vi "WiFi HttpsPOST.vi"   [LabVIEW 2014]
uses:
  <vilib>/Aledyne-TSXperts/Arduino Compatible Compiler for LabVIEW/Code Generator/Arduino APIs/Digital/PinDirection.ctl
  QwaveSys_ESP8266/QwaveSys_ESP8266.lvlib
  <vilib>/Aledyne-TSXperts/Arduino Compatible Compiler for LabVIEW/Arduino Compatible Compiler for LabVIEW.lvlib
types:
  T1 = typedef "Arduino Compatible Compiler for LabVIEW.lvlib/PinDirection.ctl" = enum16{" INPUT", "OUTPUT", " INPUT_PULLUP"}
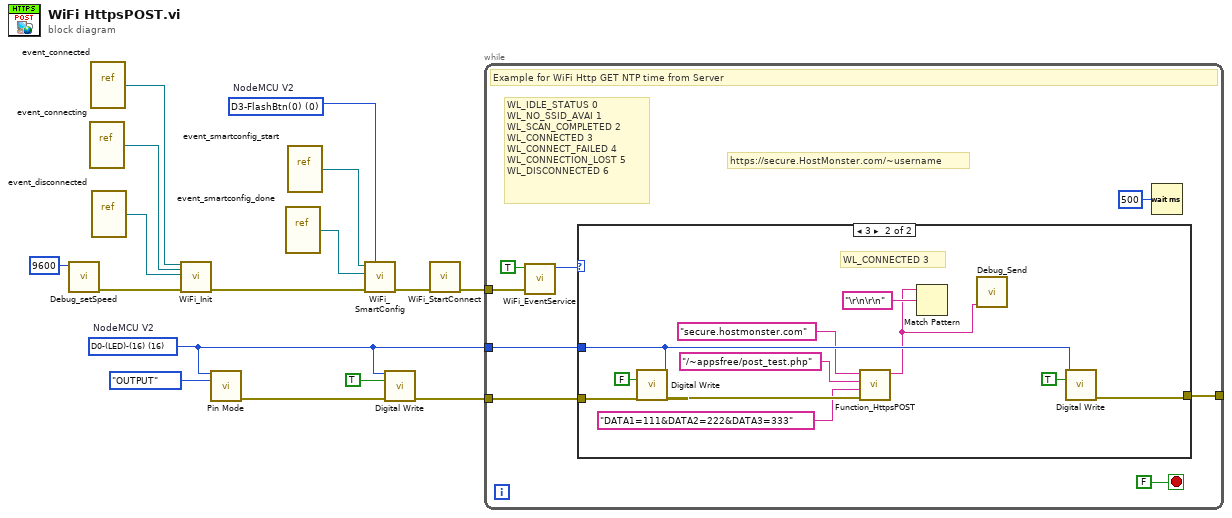
[diagram p0: block diagram]
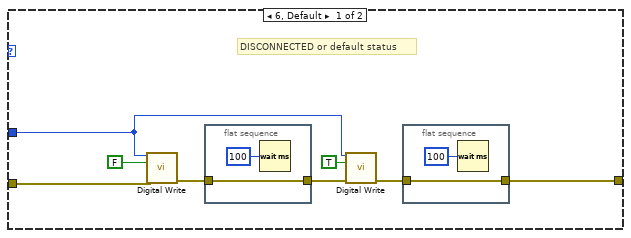
[diagram p2: hidden frame]
diagram:
  w2 = u8 16 items=["D0-(LED)-(16)"=16, "D1-SCL(5)"=5, "D2-SDA(4)"=4, "D3-FlashBtn(0)"=0, "D4-(2)"=2, "D5-SCK(14)"=14, "D6-MISO(12)"=12, "D7-MOSI(13)"=13, "D8-SS(15)"=15, "D9-TX(3)"=3, "D10-RX(1)"=1, "ADC0,(17)"=17]  # NodeMCU V2
  w1 = u8 0 items=["D0-(LED)-(16)"=16, "D1-SCL(5)"=5, "D2-SDA(4)"=4, "D3-FlashBtn(0)"=0, "D4-(2)"=2, "D5-SCK(14)"=14, "D6-MISO(12)"=12, "D7-MOSI(13)"=13, "D8-SS(15)"=15, "D9-TX(3)"=3, "D10-RX(1)"=1, "ADC0,(17)"=17]  # NodeMCU V2
  n1 = call "Debug_setSpeed.vi"("Speed"=u32 9600) -> ("error out"=w8:errorcluster)  [unwired: 10 in]
  n2 = vi-ref "event_connecting.vi"() -> (w13:refnum<vi>)
  n3 = vi-ref "event_connected.vi"() -> (w12:refnum<vi>)
  n4 = vi-ref "event_disconnected.vi"() -> (w11:refnum<vi>)
  n5 = call "WiFi_Init.vi"("connected"=w12, "connecting"=w13, "disconnected"=w11, "error in (no error)"=w8) -> ("error out"=w16:errorcluster)  [unwired: 11 in]
  n6 = call <vilib>:"Pin Mode.vi"("pin"=w2, "direction"=PinDirection."OUTPUT" ("Direction")) -> ("error out"=w4:errorcluster)  [unwired: 13 in]
  n7 = vi-ref "event_smartconfig_done.vi"() -> (w9:refnum<vi>)
  n8 = vi-ref "event_smartconfig_start.vi"() -> (w10:refnum<vi>)
  n9 = call "WiFi_SmartConfig.vi"("Smart Config Enter Pin"=w1, "error in (no error)"=w16, "smartconfig_done"=w9, "smartconfig_start"=w10) -> ("error out"=w15:errorcluster)  [unwired: 7 in]
  n10 = call <vilib>:"Digital Write.vi"("pin"=w2, "state"=TRUE, "error in (no error)"=w4) -> ("error out"=w3:errorcluster)  [unwired: 12 in]
  n11 = call "WiFi_StartConnect.vi"("error in (no error)"=w15) -> ("error out"=w14:errorcluster)  [unwired: 10 in]
  n12 = while {
    tunnel: w14 -> [w23]
    tunnel: w3 -> [w19]
    tunnel: w2 -> [w18]
    tunnel: [w17] -> _
    stop <- FALSE stop-if-true
    # "https://secure.HostMonster.com/~username"
    # "WL_IDLE_STATUS\t0\nWL_NO_SSID_AVAI\t1\nWL_SCAN_COMPLETED\t2\nWL_CONNECTED\t3\nWL_CONNECT_FAILED\t4\nWL_CONNECTION_LOST\t5\nWL_DISCONNECTED\t6"
    # "Example for WiFi Http GET NTP time from Server"
    n13 = call "WiFi_EventService.vi"("error in (no error)"=w23, "wait for connected (True)"=TRUE) -> ("Status"=w20:u16)  [unwired: 8 in, 1 out]
    n14 = case shown="3" w20 {
      tunnel: w19 -> [w27 w45]
      tunnel: w18 -> [w26 w44]
      tunnel: [w25 w42] -> w17
      frame 6, Default {
        # "DISCONNECTED or default status"
        n15 = call <vilib>:"Digital Write.vi"("pin"=w26, "state"=FALSE, "error in (no error)"=w27) -> ("error out"=w28:errorcluster)  [unwired: 12 in]
        n16 = flat-sequence {
          tunnel: w28 -> [w35]
          tunnel: [w35] -> w29
          frame #0 {
            n17 = Wait (ms)(milliseconds to wait=u32 100) -> ()  [unwired: 1 out]
          }
        }
        n18 = call <vilib>:"Digital Write.vi"("pin"=w26, "state"=TRUE, "error in (no error)"=w29) -> ("error out"=w32:errorcluster)  [unwired: 12 in]
        n19 = flat-sequence {
          tunnel: w32 -> [w33]
          tunnel: [w33] -> w25
          frame #0 {
            n20 = Wait (ms)(milliseconds to wait=u32 100) -> ()  [unwired: 1 out]
          }
        }
      }
      frame 3 {
        # "WL_CONNECTED\t3"
        n21 = call <vilib>:"Digital Write.vi"("pin"=w44, "state"=FALSE, "error in (no error)"=w45) -> ("error out"=w41:errorcluster)  [unwired: 12 in]
        n22 = call "Function_HttpsPOST.vi"("error in (no error)"=w41, "DATA"="DATA1=111&DATA2=222&DATA3=333" ("URI"), "URI"="/~appsfree/post_test.php", "Host"="secure.hostmonster.com") -> ("Results"=w37:string)  [unwired: 6 in, 1 out]
        n23 = Match Pattern(string=w37, regular expression="\r\n\r\n") -> ()  [unwired: 1 in, 4 out]
        n24 = call "Debug_Send.vi"("DATA"=w37) -> ()  [unwired: 11 in]
        n25 = call <vilib>:"Digital Write.vi"("pin"=w44, "state"=TRUE) -> ("error out"=w42:errorcluster)  [unwired: 13 in]
      }
    }
    n26 = Wait (ms)(milliseconds to wait=u32 500) -> ()  [unwired: 1 out]
  }
